vi "Close Files.vi"(8 "error in (no error)":errorcluster, 11 "CubeLogger in":refnum<class "CubeLogger.lvclass">) -> (0 "error out":errorcluster, 3 "CubeLogger out":refnum<class "CubeLogger.lvclass">)   [LabVIEW 2018, in "vis3d.lvlib" / "CubeLogger.lvclass"]
uses:
  CubeLogger.lvclass
  CubeLogger.lvclass/CubeLogger.ctl
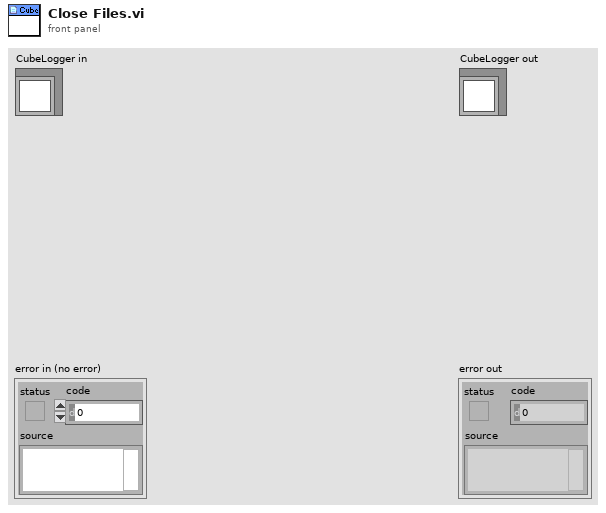
[diagram p1: front panel]
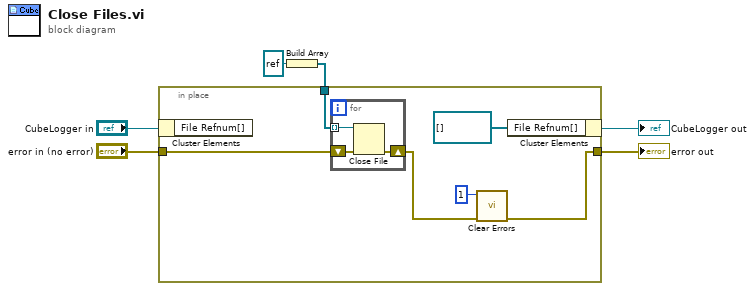
[diagram p0: block diagram]
diagram:
  n1 = Build Array(refnum<file> refnum ("File Refnum[]")) -> (w1:refnum<file>[])
  n2 = in-place {
    in-place-border: "error in (no error)" -> [w11]
    in-place-border: [w8] -> w5
    in-place-border: w1 -> [w10]
    n3 = in-place-cluster #1("CubeLogger in") -> ()  [unwired: 1 out]
    n4 = for {
      tunnel: w10 -> [w15] mode=indexing
      shift-right: [w13] -> w9
      shift-left: w11 -> [w14]
      n5 = Close File(refnum=w15, error in=w14) -> (error out=w13:errorcluster)  [unwired: 1 out]
    }
    n6 = call <vilib>:"Clear Errors.vi"("error in (no error)"=w9, "specific error code to clear (0: all)"=1) -> ("error out"=w8:errorcluster)  [unwired: 4 in, 1 out]
    n7 = in-place-cluster #1("File Refnum[]"=refnum<file>[] []) -> (→"CubeLogger out":refnum<class "CubeLogger.lvclass">)
  }
  "error out" <- w5
